vi "MotorAllInfo.vi"(3 "COM Port in":refnum<visa-resource-name>, 9 "error in (no error)":errorcluster) -> (0 "COM Port out":refnum<visa-resource-name>, 2 "Positions":i32[](array[numeric]), 6 "error out":errorcluster)   [LabVIEW 2009]
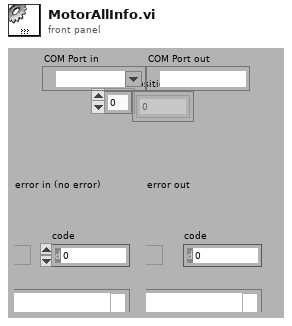
[diagram p1: front panel]
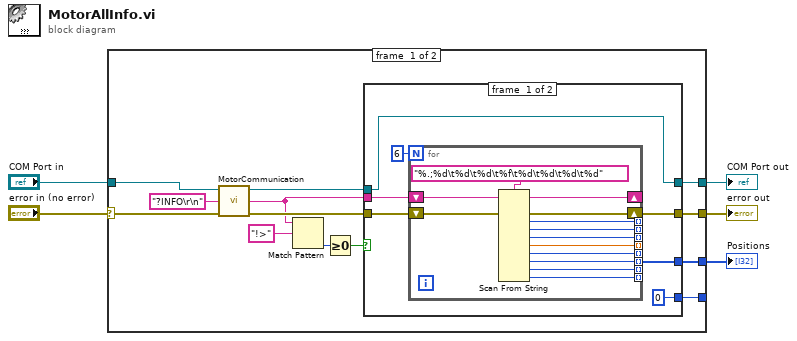
[diagram p0: block diagram]
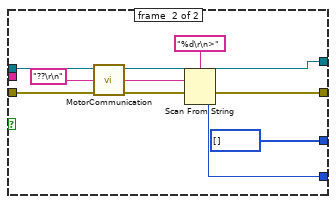
[diagram p2: hidden frame]
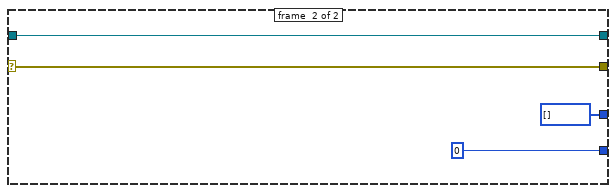
[diagram p3: hidden frame]
diagram:
  n1 = case shown="No Error" "error in (no error)" {
    selector: "error in (no error)" -> [w11 w52]
    tunnel: "COM Port in" -> [w8 w51]
    tunnel: [w17 w51] -> w2
    tunnel: [w16 w52] -> w3
    tunnel: [w13 0] -> _
    tunnel: [w12 i32[] []] -> w1
    frame #0 {
      n2 = call "MotorCommunication.vi"("Question"="?INFO\r\n", "error out"=w11, "COM Port in"=w8) -> ("error IO"=w10:errorcluster, "COM Port out"=w9:refnum<visa-resource-name>, "Answer"=w6:string)  [unwired: 4 out]
      n3 = Match Pattern(string=w6, regular expression="!>") -> (offset past match=w18:i32)  [unwired: 4 out]
      n4 = Greater Or Equal To 0?(x=w18) -> (x >= 0?=w14:bool)
      n5 = case "Structure Condition" shown="True" w14 {
        tunnel: w10 -> [w22 w44]
        tunnel: w9 -> [w20 w43]
        tunnel: [w21 w47] -> w16
        tunnel: [w20 w39] -> w17
        tunnel: [0 w46] -> w13
        tunnel: w6 -> [w24 _]
        tunnel: [w19 i32[] []] -> w12
        frame #0 {
          n6 = for {
            N: 6 -> [_]
            shift-right: [w37] -> _
            shift-left: w24 -> [w38]
            shift-right: [w34] -> w21
            shift-left: w22 -> [w35]
            tunnel: [w33] -> _ mode=indexing
            tunnel: [w32] -> _ mode=indexing
            tunnel: [w31] -> _ mode=indexing
            tunnel: [w30] -> _ mode=indexing
            tunnel: [w29] -> _ mode=indexing
            tunnel: [w28] -> w19 mode=indexing
            tunnel: [w27] -> _ mode=indexing
            tunnel: [w26] -> _ mode=indexing
            n7 = Scan From String(format string="%.;%d\t%d\t%d\t%f\t%d\t%d\t%d\t%d" ("chaîne de format"), input string=w38, error in=w35) -> (remaining string=w37:string, error out=w34:errorcluster, output 1=w33:i32, output 2=w32:i32, output 3=w31:i32, output 4=w30:dbl, output 5=w29:i32, output 6=w28:i32, output 7=w27:i32, output 8=w26:i32)  [unwired: 1 in, 9 out]
          }
        }
        frame #1 {
          n8 = call "MotorCommunication.vi"("Question"="??\r\n" ("buffer à écrire"), "error out"=w44, "COM Port in"=w43) -> ("error IO"=w40:errorcluster, "COM Port out"=w39:refnum<visa-resource-name>, "Answer"=w41:string)  [unwired: 4 out]
          n9 = Scan From String(format string="%d\r\n>" ("chaîne de format"), input string=w41, error in=w40) -> (error out=w47:errorcluster, output 1=w46:i32)  [unwired: 1 in, 3 out]
        }
      }
    }
    frame #1 {
    }
  }
  "Positions" <- w1
  "error out" <- w3
  "COM Port out" <- w2
